vi "HighShift.vi"(11 "High":bool) -> ()   [LabVIEW 2017]
uses:
  <vilib>/Rock Robotics/WPI/Solenoid/Deprecated/WPI_SolenoidSetBool.vi
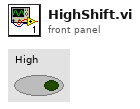
[diagram p1: front panel]
types:
  T1 = typedef "WPI_SolenoidDevRef.ctl" = cluster{"DevStatus":errorcluster, "Pneumatics Control Module":u8, "Forward Solenoid Channel":T2, "Reverse Solenoid Channel":T2}
  T2 = typedef "WPI_SolenoidChannel.ctl" = enum8{"Solenoid 0", "Solenoid 1", "Solenoid 2", "Solenoid 3", "Solenoid 4", "Solenoid 5", "Solenoid 6", "Solenoid 7", "Invalid"}
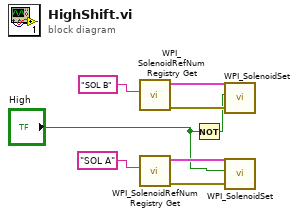
[diagram p0: block diagram]
diagram:
  n1 = call <vilib>:"WPI_SolenoidRefNum Registry Get.vi"("refnum name"="SOL B") -> ("error out"=w4:errorcluster, "SolenoidDevRef"=w3:T1)  [unwired: 9 in]
  n2 = call <vilib>:"WPI_SolenoidRefNum Registry Get.vi"("refnum name"="SOL A") -> ("error out"=w7:errorcluster, "SolenoidDevRef"=w6:T1)  [unwired: 9 in]
  n3 = Not(x="High") -> (.not. x?=w2:bool)
  n4 = call-poly <vilib>:"WPI_SolenoidSet.vi"("error in (no error)"=w4, "Value"=w2, "SolenoidDevRef"=w3) -> ()  [unwired: 7 in, 2 out]
  n5 = call-poly <vilib>:"WPI_SolenoidSet.vi"("error in (no error)"=w7, "Value"="High", "SolenoidDevRef"=w6) -> ()  [unwired: 7 in, 2 out]
